vi "measure_rotary_stage_speed.vi"(1 "Stop/Start":bool, 2 "starting edge":i32(ring)=10280 items=["Rising"=10280, "Falling"=10171], 3 "rotary out":tag, 4 "counter channel":tag="Dev1/ctr0") -> (0 "stage speed":dbl caption="actual speed(rps)" format="%0.4f")   [LabVIEW 2019]
uses:
  <vilib>/DAQmx/read.llb/DAQmx Read (Counter DBL 1Chan 1Samp).vi
  <vilib>/DAQmx/create/channels.llb/DAQmx Create Channel (CI-Frequency).vi
  <vilib>/DAQmx/miscellaneous.llb/DAQmx Fill In Error Info.vi
  <resource>/objmgr/daqmx.rc
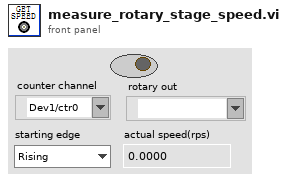
[diagram p1: front panel]
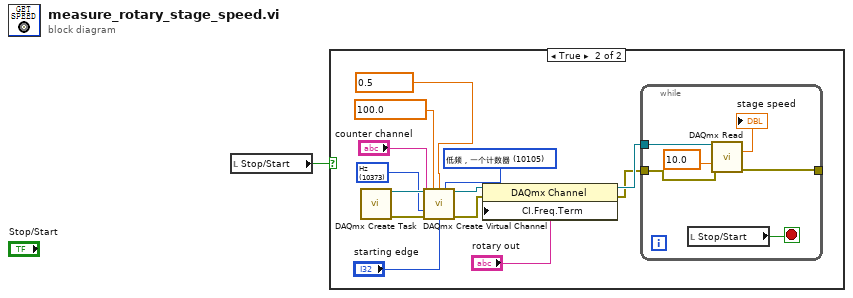
[diagram p0: block diagram]
diagram:
  n1 = local read "Stop/Start"() -> (w1:bool)
  n2 = case shown="True" w1 {
    frame False {
    }
    frame True {
      w9 = 10105 items=["低频，一个计数器"=10105, "高频，两个计数器"=10157, "大范围，两个计数器"=10205, "动态均值"=16065] ("measurement method")
      w8 = 10373 items=["Hz"=10373, "时钟滴答"=10304, "来自自定义换算"=10065] ("units")
      n3 = call <vilib>:"DAQmx Create Task.vi"() -> ("task out"=w12:refnum<k21>, "error out"=w13:errorcluster)  [unwired: 14 in]
      n4 = call-poly <vilib>:"DAQmx Create Virtual Channel.vi"("task in"=w12, "maximum value"=100.0, "minimum value"=0.5, "measurement method"=w9, "counter"="counter channel", "units"=w8, "error in"=w13, "starting edge"="starting edge") -> ("task out"=w6:refnum<k21>, "error out"=w5:errorcluster)  [unwired: 6 in]
      n5 = property class="DAQmx Channel"(reference=w6, error in=w5, "CI.Freq.Term"="rotary out") -> (reference out=w3:refnum<k21>, error out=w2:errorcluster)
      n6 = while {
        tunnel: w3 -> [w20]
        tunnel: w2 -> [w19]
        tunnel: [w17] -> _
        stop <- w15 stop-if-true
        n7 = local read "Stop/Start"() -> (w15:bool)
        n8 = call-poly <vilib>:"DAQmx Read.vi"("task/channels in"=w20, "timeout"=10.0 ("timeout (s)"), "error in"=w19) -> ("data"=→"stage speed":dbl, "error out"=w17:errorcluster)  [unwired: 10 in, 1 out]
      }
    }
  }
